vi "OpenSVConnectionInBG.vi"(8 "error in (no error)":errorcluster, 9 "ChannelNames":string[](array[string]), 10 "Target IP":string, 11 "DeviceName":string) -> (0 "error out":errorcluster, 3 "SharedVariableRefnums":refnum<k21>[](array[refnum]))   [LabVIEW 2013]
uses:
  AI_Data.ctl
  NI Card.lvclass
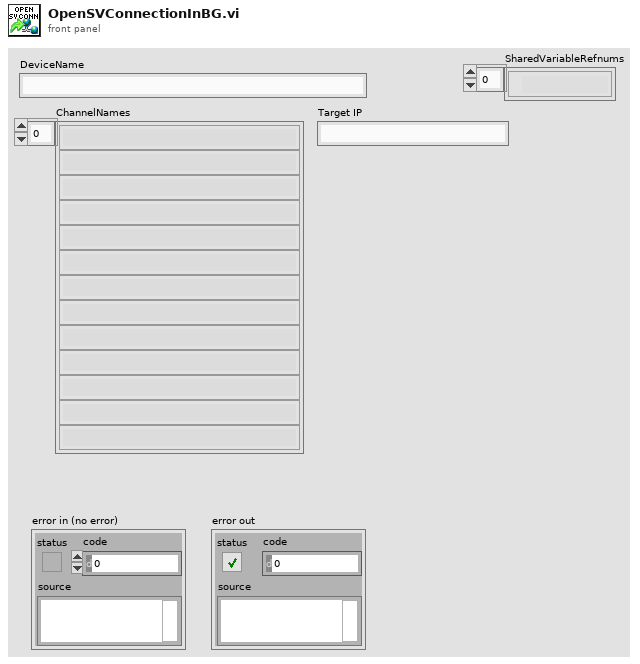
[diagram p1: front panel]
types:
  T1 = cluster{"Read Access":enum8{"Allowed", "Required", "None"}, "Write Access":enum8{"Allowed", "Required", "None"}}
  T2 = typedef "NI Card.lvclass/AI_Data.ctl" = cluster{"dt":dbl, "y":dbl[], "Channel Name":string, "FileNum":u32}
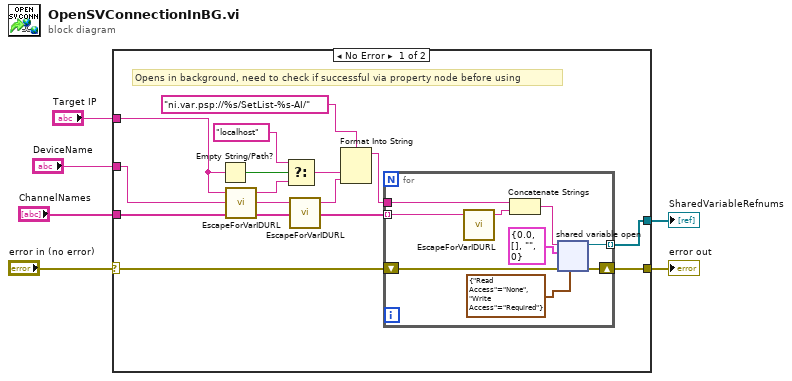
[diagram p0: block diagram]
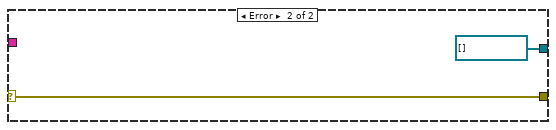
[diagram p2: hidden frame]
diagram:
  n1 = case shown="No Error" "error in (no error)" {
    selector: "error in (no error)" -> [w12 w30]
    tunnel: "DeviceName" -> [w19 _]
    tunnel: "Target IP" -> [w8 _]
    tunnel: "ChannelNames" -> [w15 _]
    tunnel: [w14 refnum<k21>[] []] -> w3
    tunnel: [w13 w30] -> w2
    frame No Error {
      # "Opens in background, need to check if successful via property node before using"
      n2 = Empty String/Path?(string/path=w8) -> (empty?=w10:bool)
      n3 = call "EscapeForVarIDURL.vi"("Unescaped String"=w8) -> ("VarID URL String"=w7:string)  [unwired: 4 in]
      n4 = Select(t="localhost", s=w10, f=w7) -> (s? t:f=w9:string)
      n5 = call "EscapeForVarIDURL.vi"("Unescaped String"=w19) -> ("VarID URL String"=w18:string)  [unwired: 4 in]
      n6 = Format Into String(format string="ni.var.psp://%s/SetList-%s-AI/", w9, w18) -> (resulting string=w16:string)  [unwired: 2 in, 1 out]
      n7 = for {
        tunnel: w16 -> [w26]
        tunnel: w15 -> [w28] mode=indexing
        shift-right: [w21] -> w13
        shift-left: w12 -> [w22]
        tunnel: [w20] -> w14 mode=indexing
        n8 = call "EscapeForVarIDURL.vi"("Unescaped String"=w28) -> ("VarID URL String"=w27:string)  [unwired: 4 in]
        n9 = Concatenate Strings(w26, w27) -> (w24:string)
        n10 = shared-variable-open(w24, w22, T2 {"dt"=0.0, "y"=[], "Channel Name"="", "FileNum"=0} ("AI Data"), T1 {"Read Access"=enum."None", "Write Access"=enum."Required"} ("access")) -> (w20:refnum<k21>, w21:errorcluster)  [unwired: 1 in]
      }
    }
    frame Error {
    }
  }
  "error out" <- w2
  "SharedVariableRefnums" <- w3
